vi "readTelemetryForceActuatorStatus.vi"(8 "error in (no error)":errorcluster, 10 "Parser":refnum<class "U8ArrayParserAutoIndexing.lvclass">, 11 "M1M3SAL in":refnum<class "M1M3SAL.lvclass">) -> (0 "error out":errorcluster, 2 "EventSummaryState":variant, 3 "M1M3SAL out":refnum<class "M1M3SAL.lvclass">)   [LabVIEW 2016, in "M1M3SupportCommunicator.lvlib" / "M1M3SAL.lvclass"]
uses:
  M1M3SAL.lvclass
  Common_RT_Utilities/U8ArrayParserAutoIndexing/U8ArrayParserAutoIndexing.lvclass
  DataTypes/Topics/TelemetryForceActuatorStatus.ctl
  DataTypes/Topics/Parts/Timestamp.ctl
  DataTypes/Topics/M1M3SupportTopics.lvlib
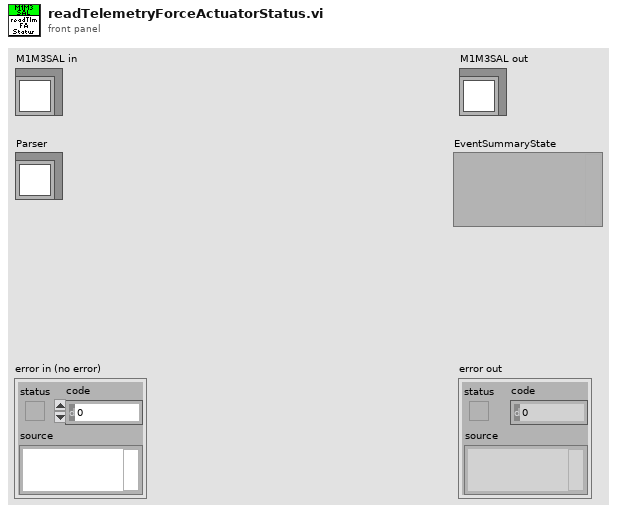
[diagram p1: front panel]
types:
  T1 = typedef "M1M3SupportTopics.lvlib/TelemetryForceActuatorStatus.ctl" = cluster{"Timestamp":T2, "Mode":u8[], "MajorFault":bool[], "MinorFault":bool[], "FaultOverridden":bool[], "DCAFault":bool[], "WatchdogReset":bool[], "BrownoutDetected":bool[], "EventTrapReset":bool[], "MotorPowerFault":bool[], "SSRPowerFault":bool[], "AUXPowerFault":bool[], "SMCPowerFault":bool[], "DCAOutputsEnabled":bool[], "DCAPowerFault":bool[], "DCAAmplifierAFault":bool[], "DCAAmplifierBFault":bool[], "DCAEventTrapReset":bool[]}
  T2 = typedef "M1M3SupportTopics.lvlib/Timestamp.ctl" = dbl
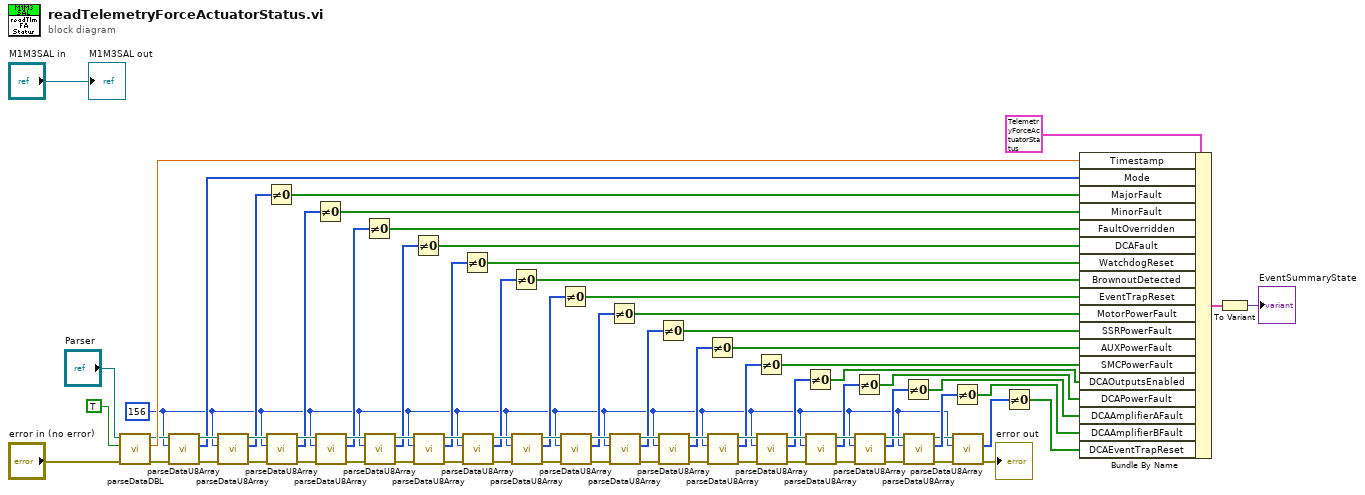
[diagram p0: block diagram]
diagram:
  w2 = 156 ("Length")
  n1 = call "parseDataDBL.vi"("error in (no error)"="error in (no error)", "OverrideSwapBytes"=TRUE, "U8ArrayParserAutoIndexing in"="Parser") -> ("error out"=w45:errorcluster, "Data"=w72:dbl, "U8ArrayParserAutoIndexing out"=w46:refnum<class "U8ArrayParserAutoIndexing.lvclass">)  [unwired: 6 in]
  n2 = call "parseDataU8Array.vi"("U8ArrayParserAutoIndexing in"=w46, "Length"=w2, "error in (no error)"=w45) -> ("U8ArrayParserAutoIndexing out"=w70:refnum<class "U8ArrayParserAutoIndexing.lvclass">, "Data"=w38:u8[], "error out"=w69:errorcluster)  [unwired: 5 in]
  n3 = call "parseDataU8Array.vi"("U8ArrayParserAutoIndexing in"=w70, "Length"=w2, "error in (no error)"=w69) -> ("U8ArrayParserAutoIndexing out"=w68:refnum<class "U8ArrayParserAutoIndexing.lvclass">, "Data"=w37:u8[], "error out"=w67:errorcluster)  [unwired: 5 in]
  n4 = Not Equal To 0?(x=w37) -> (x != 0?=w36:bool[])
  n5 = call "parseDataU8Array.vi"("U8ArrayParserAutoIndexing in"=w68, "Length"=w2, "error in (no error)"=w67) -> ("U8ArrayParserAutoIndexing out"=w44:refnum<class "U8ArrayParserAutoIndexing.lvclass">, "Data"=w35:u8[], "error out"=w43:errorcluster)  [unwired: 5 in]
  n6 = Not Equal To 0?(x=w35) -> (x != 0?=w34:bool[])
  n7 = call "parseDataU8Array.vi"("U8ArrayParserAutoIndexing in"=w44, "Length"=w2, "error in (no error)"=w43) -> ("U8ArrayParserAutoIndexing out"=w42:refnum<class "U8ArrayParserAutoIndexing.lvclass">, "Data"=w33:u8[], "error out"=w41:errorcluster)  [unwired: 5 in]
  n8 = Not Equal To 0?(x=w33) -> (x != 0?=w32:bool[])
  n9 = call "parseDataU8Array.vi"("U8ArrayParserAutoIndexing in"=w42, "Length"=w2, "error in (no error)"=w41) -> ("U8ArrayParserAutoIndexing out"=w66:refnum<class "U8ArrayParserAutoIndexing.lvclass">, "Data"=w31:u8[], "error out"=w65:errorcluster)  [unwired: 5 in]
  n10 = Not Equal To 0?(x=w31) -> (x != 0?=w30:bool[])
  n11 = call "parseDataU8Array.vi"("U8ArrayParserAutoIndexing in"=w66, "Length"=w2, "error in (no error)"=w65) -> ("U8ArrayParserAutoIndexing out"=w64:refnum<class "U8ArrayParserAutoIndexing.lvclass">, "Data"=w29:u8[], "error out"=w63:errorcluster)  [unwired: 5 in]
  n12 = Not Equal To 0?(x=w29) -> (x != 0?=w28:bool[])
  n13 = call "parseDataU8Array.vi"("U8ArrayParserAutoIndexing in"=w64, "Length"=w2, "error in (no error)"=w63) -> ("U8ArrayParserAutoIndexing out"=w62:refnum<class "U8ArrayParserAutoIndexing.lvclass">, "Data"=w27:u8[], "error out"=w61:errorcluster)  [unwired: 5 in]
  n14 = Not Equal To 0?(x=w27) -> (x != 0?=w26:bool[])
  n15 = call "parseDataU8Array.vi"("U8ArrayParserAutoIndexing in"=w62, "Length"=w2, "error in (no error)"=w61) -> ("U8ArrayParserAutoIndexing out"=w60:refnum<class "U8ArrayParserAutoIndexing.lvclass">, "Data"=w25:u8[], "error out"=w59:errorcluster)  [unwired: 5 in]
  n16 = Not Equal To 0?(x=w25) -> (x != 0?=w24:bool[])
  n17 = call "parseDataU8Array.vi"("U8ArrayParserAutoIndexing in"=w60, "Length"=w2, "error in (no error)"=w59) -> ("U8ArrayParserAutoIndexing out"=w58:refnum<class "U8ArrayParserAutoIndexing.lvclass">, "Data"=w23:u8[], "error out"=w57:errorcluster)  [unwired: 5 in]
  n18 = Not Equal To 0?(x=w23) -> (x != 0?=w22:bool[])
  n19 = call "parseDataU8Array.vi"("U8ArrayParserAutoIndexing in"=w58, "Length"=w2, "error in (no error)"=w57) -> ("U8ArrayParserAutoIndexing out"=w40:refnum<class "U8ArrayParserAutoIndexing.lvclass">, "Data"=w21:u8[], "error out"=w39:errorcluster)  [unwired: 5 in]
  n20 = Not Equal To 0?(x=w21) -> (x != 0?=w20:bool[])
  n21 = call "parseDataU8Array.vi"("U8ArrayParserAutoIndexing in"=w40, "Length"=w2, "error in (no error)"=w39) -> ("U8ArrayParserAutoIndexing out"=w56:refnum<class "U8ArrayParserAutoIndexing.lvclass">, "Data"=w19:u8[], "error out"=w55:errorcluster)  [unwired: 5 in]
  n22 = Not Equal To 0?(x=w19) -> (x != 0?=w18:bool[])
  n23 = call "parseDataU8Array.vi"("U8ArrayParserAutoIndexing in"=w56, "Length"=w2, "error in (no error)"=w55) -> ("U8ArrayParserAutoIndexing out"=w54:refnum<class "U8ArrayParserAutoIndexing.lvclass">, "Data"=w17:u8[], "error out"=w53:errorcluster)  [unwired: 5 in]
  n24 = Not Equal To 0?(x=w17) -> (x != 0?=w16:bool[])
  n25 = call "parseDataU8Array.vi"("U8ArrayParserAutoIndexing in"=w54, "Length"=w2, "error in (no error)"=w53) -> ("U8ArrayParserAutoIndexing out"=w52:refnum<class "U8ArrayParserAutoIndexing.lvclass">, "Data"=w15:u8[], "error out"=w51:errorcluster)  [unwired: 5 in]
  n26 = Not Equal To 0?(x=w15) -> (x != 0?=w14:bool[])
  n27 = call "parseDataU8Array.vi"("U8ArrayParserAutoIndexing in"=w52, "Length"=w2, "error in (no error)"=w51) -> ("U8ArrayParserAutoIndexing out"=w50:refnum<class "U8ArrayParserAutoIndexing.lvclass">, "Data"=w13:u8[], "error out"=w49:errorcluster)  [unwired: 5 in]
  n28 = Not Equal To 0?(x=w13) -> (x != 0?=w12:bool[])
  n29 = call "parseDataU8Array.vi"("U8ArrayParserAutoIndexing in"=w50, "Length"=w2, "error in (no error)"=w49) -> ("U8ArrayParserAutoIndexing out"=w48:refnum<class "U8ArrayParserAutoIndexing.lvclass">, "Data"=w11:u8[], "error out"=w47:errorcluster)  [unwired: 5 in]
  n30 = Not Equal To 0?(x=w11) -> (x != 0?=w10:bool[])
  n31 = call "parseDataU8Array.vi"("U8ArrayParserAutoIndexing in"=w48, "Length"=w2, "error in (no error)"=w47) -> ("U8ArrayParserAutoIndexing out"=w8:refnum<class "U8ArrayParserAutoIndexing.lvclass">, "Data"=w9:u8[], "error out"=w7:errorcluster)  [unwired: 5 in]
  n32 = Not Equal To 0?(x=w9) -> (x != 0?=w3:bool[])
  n33 = call "parseDataU8Array.vi"("U8ArrayParserAutoIndexing in"=w8, "Length"=w2, "error in (no error)"=w7) -> ("Data"=w5:u8[], "error out"=→"error out":errorcluster)  [unwired: 5 in, 1 out]
  n34 = Not Equal To 0?(x=w5) -> (x != 0?=w4:bool[])
  n35 = Bundle By Name(cluster=T1 {"Timestamp"=0.0, "Mode"=[], "MajorFault"=[], "MinorFault"=[], "FaultOverridden"=[], "DCAFault"=[], "WatchdogReset"=[], "BrownoutDetected"=[], "EventTrapReset"=[], "MotorPowerFault"=[], "SSRPowerFault"=[], "AUXPowerFault"=[], "SMCPowerFault"=[], "DCAOutputsEnabled"=[], "DCAPowerFault"=[], "DCAAmplifierAFault"=[], "DCAAmplifierBFault"=[], "DCAEventTrapReset"=[]} ("TelemetryForceActuatorStatus"), "Timestamp"=w72, "Mode"=w38, "MajorFault"=w36, "MinorFault"=w34, "FaultOverridden"=w32, "DCAFault"=w30, "WatchdogReset"=w28, "BrownoutDetected"=w26, "EventTrapReset"=w24, "MotorPowerFault"=w22, "SSRPowerFault"=w20, "AUXPowerFault"=w18, "SMCPowerFault"=w16, "DCAOutputsEnabled"=w14, "DCAPowerFault"=w12, "DCAAmplifierAFault"=w10, "DCAAmplifierBFault"=w3, "DCAEventTrapReset"=w4) -> (w76:T1)
  n36 = To Variant(anything=w76) -> (Variant=→"EventSummaryState":variant)
  "M1M3SAL out" <- "M1M3SAL in"
